vi "Set ch (SubVI).vi"(8 "2400通道":i32, 9 "initialize":T1, 10 "数值":i32, 11 "Instrument Type":T2=enum."PPMS-Rotate") -> ()   [LabVIEW 2019, in "SubVI.lvlib"]
uses:
  SubVI.lvlib
  ctl/Instrument Type.ctl
  ctl/initialize.ctl
  lib/KE7001.LLB/Keith 7001 Open/Close Chan.vi
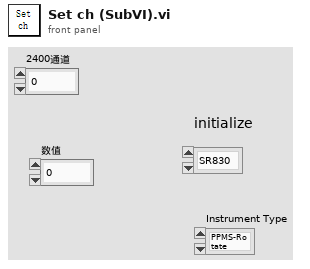
[diagram p1: front panel]
types:
  T1 = typedef "initialize.ctl" = enum16{"SR830", "keithley6221-SR830", "Delta", "Delta-tunnelling", "keithley6221-2182-DC", "PZT", "StrainCell", "4200"}
  T2 = typedef "Instrument Type.ctl" = enum16{"PPMS", "VersaLab", "DynaCool", "SVSM", "PPMS-Rotate", "Lakeshore335", "2T cmag", "9T mag old", "9T cmag", "9T cmag DAC", "9T cmag rotate", "test"}
  T3 = cluster{"slot/memory":i16, "channel/row":i16, "column":i16, bool, bool}[]
  T4 = cluster{"error":bool, "code":i32, "source":string}
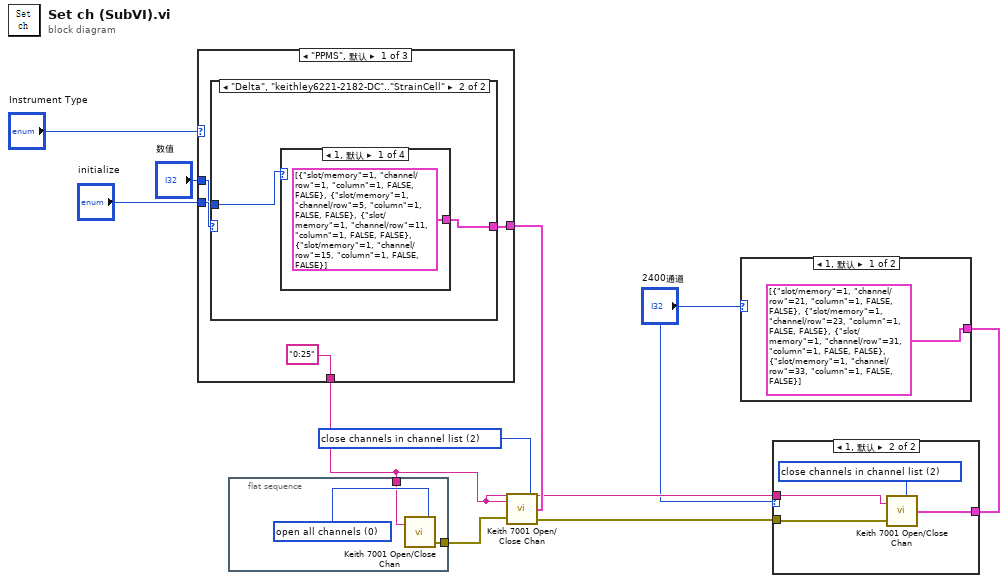
[diagram p0: block diagram]
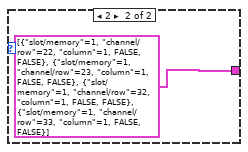
[diagram p2: hidden frame]
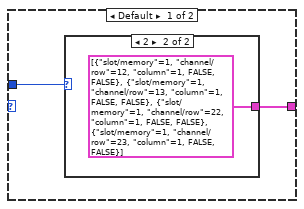
[diagram p4: hidden frame]
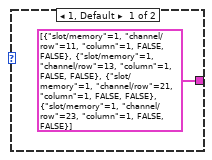
[diagram p5: hidden frame]
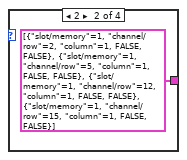
[diagram p6: hidden frame]
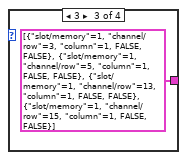
[diagram p7: hidden frame]
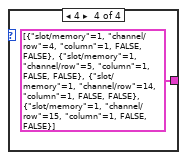
[diagram p8: hidden frame]
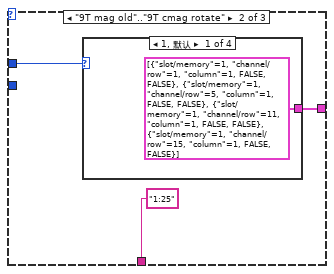
[diagram p9: hidden frame]
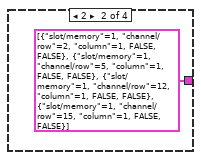
[diagram p10: hidden frame]
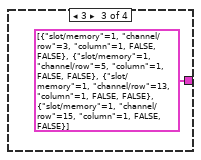
[diagram p11: hidden frame]
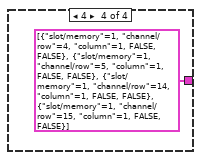
[diagram p12: hidden frame]
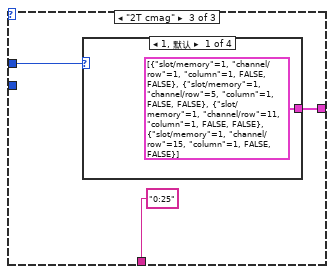
[diagram p13: hidden frame]
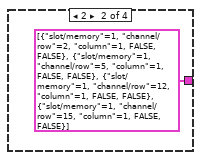
[diagram p14: hidden frame]
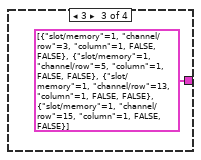
[diagram p15: hidden frame]
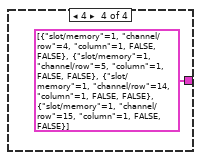
[diagram p16: hidden frame]
diagram:
  w10 = u16 2 items=["open all channels", "open channels in channel list", "close channels in channel list"] ("open/close (open all:0)")
  n1 = case shown="\"PPMS\", 默认" "Instrument Type" {
    tunnel: [w14 w26 w33] -> w8
    tunnel: "initialize" -> [w13 _ _]
    tunnel: "数值" -> [w12 w27 w34]
    tunnel: ["0:25" ("GPIB address") "1:25" ("GPIB address") "0:25" ("GPIB address")] -> w4
    frame "PPMS", Default {
      n2 = case shown="\"Delta\", \"keithley6221-2182-DC\"..\"StrainCell\"" w13 {
        tunnel: [w16 w20] -> w14
        tunnel: w12 -> [w15 w19]
        frame Default {
          n3 = case shown="2" w15 {
            tunnel: [T3 [{"slot/memory"=1, "channel/row"=11, "column"=1, FALSE, FALSE}, {"slot/memory"=1, "channel/row"=13, "column"=1, FALSE, FALSE}, {"slot/memory"=1, "channel/row"=21, "column"=1, FALSE, FALSE}, {"slot/memory"=1, "channel/row"=23, "column"=1, FALSE, FALSE}] ("channel list") T3 [{"slot/memory"=1, "channel/row"=12, "column"=1, FALSE, FALSE}, {"slot/memory"=1, "channel/row"=13, "column"=1, FALSE, FALSE}, {"slot/memory"=1, "channel/row"=22, "column"=1, FALSE, FALSE}, {"slot/memory"=1, "channel/row"=23, "column"=1, FALSE, FALSE}] ("channel list")] -> w16
            frame 1, Default {
            }
            frame 2 {
            }
          }
        }
        frame "Delta", "keithley6221-2182-DC".."StrainCell" {
          n4 = case shown="1, 默认" w19 {
            tunnel: [T3 [{"slot/memory"=1, "channel/row"=1, "column"=1, FALSE, FALSE}, {"slot/memory"=1, "channel/row"=5, "column"=1, FALSE, FALSE}, {"slot/memory"=1, "channel/row"=11, "column"=1, FALSE, FALSE}, {"slot/memory"=1, "channel/row"=15, "column"=1, FALSE, FALSE}] ("channel list") T3 [{"slot/memory"=1, "channel/row"=2, "column"=1, FALSE, FALSE}, {"slot/memory"=1, "channel/row"=5, "column"=1, FALSE, FALSE}, {"slot/memory"=1, "channel/row"=12, "column"=1, FALSE, FALSE}, {"slot/memory"=1, "channel/row"=15, "column"=1, FALSE, FALSE}] ("channel list") T3 [{"slot/memory"=1, "channel/row"=3, "column"=1, FALSE, FALSE}, {"slot/memory"=1, "channel/row"=5, "column"=1, FALSE, FALSE}, {"slot/memory"=1, "channel/row"=13, "column"=1, FALSE, FALSE}, {"slot/memory"=1, "channel/row"=15, "column"=1, FALSE, FALSE}] ("channel list") T3 [{"slot/memory"=1, "channel/row"=4, "column"=1, FALSE, FALSE}, {"slot/memory"=1, "channel/row"=5, "column"=1, FALSE, FALSE}, {"slot/memory"=1, "channel/row"=14, "column"=1, FALSE, FALSE}, {"slot/memory"=1, "channel/row"=15, "column"=1, FALSE, FALSE}] ("channel list")] -> w20
            frame 1, Default {
            }
            frame 2 {
            }
            frame 3 {
            }
            frame 4 {
            }
          }
        }
      }
    }
    frame "9T mag old".."9T cmag rotate" {
      n5 = case shown="1, 默认" w27 {
        tunnel: [T3 [{"slot/memory"=1, "channel/row"=1, "column"=1, FALSE, FALSE}, {"slot/memory"=1, "channel/row"=5, "column"=1, FALSE, FALSE}, {"slot/memory"=1, "channel/row"=11, "column"=1, FALSE, FALSE}, {"slot/memory"=1, "channel/row"=15, "column"=1, FALSE, FALSE}] ("channel list") T3 [{"slot/memory"=1, "channel/row"=2, "column"=1, FALSE, FALSE}, {"slot/memory"=1, "channel/row"=5, "column"=1, FALSE, FALSE}, {"slot/memory"=1, "channel/row"=12, "column"=1, FALSE, FALSE}, {"slot/memory"=1, "channel/row"=15, "column"=1, FALSE, FALSE}] ("channel list") T3 [{"slot/memory"=1, "channel/row"=3, "column"=1, FALSE, FALSE}, {"slot/memory"=1, "channel/row"=5, "column"=1, FALSE, FALSE}, {"slot/memory"=1, "channel/row"=13, "column"=1, FALSE, FALSE}, {"slot/memory"=1, "channel/row"=15, "column"=1, FALSE, FALSE}] ("channel list") T3 [{"slot/memory"=1, "channel/row"=4, "column"=1, FALSE, FALSE}, {"slot/memory"=1, "channel/row"=5, "column"=1, FALSE, FALSE}, {"slot/memory"=1, "channel/row"=14, "column"=1, FALSE, FALSE}, {"slot/memory"=1, "channel/row"=15, "column"=1, FALSE, FALSE}] ("channel list")] -> w26
        frame 1, Default {
        }
        frame 2 {
        }
        frame 3 {
        }
        frame 4 {
        }
      }
    }
    frame "2T cmag" {
      n6 = case shown="1, 默认" w34 {
        tunnel: [T3 [{"slot/memory"=1, "channel/row"=1, "column"=1, FALSE, FALSE}, {"slot/memory"=1, "channel/row"=5, "column"=1, FALSE, FALSE}, {"slot/memory"=1, "channel/row"=11, "column"=1, FALSE, FALSE}, {"slot/memory"=1, "channel/row"=15, "column"=1, FALSE, FALSE}] ("channel list") T3 [{"slot/memory"=1, "channel/row"=2, "column"=1, FALSE, FALSE}, {"slot/memory"=1, "channel/row"=5, "column"=1, FALSE, FALSE}, {"slot/memory"=1, "channel/row"=12, "column"=1, FALSE, FALSE}, {"slot/memory"=1, "channel/row"=15, "column"=1, FALSE, FALSE}] ("channel list") T3 [{"slot/memory"=1, "channel/row"=3, "column"=1, FALSE, FALSE}, {"slot/memory"=1, "channel/row"=5, "column"=1, FALSE, FALSE}, {"slot/memory"=1, "channel/row"=13, "column"=1, FALSE, FALSE}, {"slot/memory"=1, "channel/row"=15, "column"=1, FALSE, FALSE}] ("channel list") T3 [{"slot/memory"=1, "channel/row"=4, "column"=1, FALSE, FALSE}, {"slot/memory"=1, "channel/row"=5, "column"=1, FALSE, FALSE}, {"slot/memory"=1, "channel/row"=14, "column"=1, FALSE, FALSE}, {"slot/memory"=1, "channel/row"=15, "column"=1, FALSE, FALSE}] ("channel list")] -> w33
        frame 1, Default {
        }
        frame 2 {
        }
        frame 3 {
        }
        frame 4 {
        }
      }
    }
  }
  n7 = flat-sequence {
    tunnel: [w40] -> w9
    tunnel: w4 -> [w39]
    frame #0 {
      w41 = u16 0 items=["open all channels", "open channels in channel list", "close channels in channel list"] ("open/close (open all:0)")
      n8 = call "Keith 7001 Open/Close Chan.vi"("GPIB address"=w39, "open/close (open all:0)"=w41) -> ("error out"=w40:T4)  [unwired: 2 in]
    }
  }
  n9 = call "Keith 7001 Open/Close Chan.vi"("GPIB address"=w4, "error in"=w9, "open/close (open all:0)"=w10, "channel list"=w8) -> ("error out"=w5:T4)
  n10 = case shown="1, 默认" "2400通道" {
    tunnel: [T3 [{"slot/memory"=1, "channel/row"=21, "column"=1, FALSE, FALSE}, {"slot/memory"=1, "channel/row"=23, "column"=1, FALSE, FALSE}, {"slot/memory"=1, "channel/row"=31, "column"=1, FALSE, FALSE}, {"slot/memory"=1, "channel/row"=33, "column"=1, FALSE, FALSE}] ("channel list") T3 [{"slot/memory"=1, "channel/row"=22, "column"=1, FALSE, FALSE}, {"slot/memory"=1, "channel/row"=23, "column"=1, FALSE, FALSE}, {"slot/memory"=1, "channel/row"=32, "column"=1, FALSE, FALSE}, {"slot/memory"=1, "channel/row"=33, "column"=1, FALSE, FALSE}] ("channel list")] -> w6
    frame 1, Default {
    }
    frame 2 {
    }
  }
  n11 = case shown="1, 默认" "2400通道" {
    tunnel: w6 -> [_ w47]
    tunnel: w5 -> [_ w46]
    tunnel: w4 -> [_ w45]
    frame 0 {
    }
    frame 1, Default {
      w44 = u16 2 items=["open all channels", "open channels in channel list", "close channels in channel list"] ("open/close (open all:0)")
      n12 = call "Keith 7001 Open/Close Chan.vi"("GPIB address"=w45, "error in"=w46, "open/close (open all:0)"=w44, "channel list"=w47) -> ()  [unwired: 1 out]
    }
  }
